vi "FPGA tester.vi"(4 "error in":errorcluster, 6 "Repetitions":dbl=1.0, 7 "Levels":i16[](array[numeric])) -> (0 "Error out":errorcluster[][](array[cluster]), 3 "Results":dbl[][](array[numeric]))   [LabVIEW 2013]
uses:
  <vilib>/DAQmx/read.llb/DAQmx Read (Counter DBL 1Chan 1Samp).vi
  <vilib>/DAQmx/write.llb/DAQmx Write (Digital Bool 1Line 1Point).vi
  <vilib>/DAQmx/read.llb/DAQmx Read (Digital Bool 1Line 1Point).vi
  <vilib>/Utility/file.llb/Read From Spreadsheet File (I64).vi
  <vilib>/DAQmx/create/channels.llb/DAQmx Create Channel (CI-Pulse Width).vi
  <vilib>/DAQmx/miscellaneous.llb/DAQmx Fill In Error Info.vi
  <vilib>/Utility/file.llb/Write To Spreadsheet File (DBL).vi
  <resource>/objmgr/daqmx.rc
panel:
  in  "Delay":u32
  in  "GPIB address":string="15"
  in  "Write to file?":bool
  out "Trial time vs. photons counted":cluster{"Y":dbl[], "Y":dbl[]}[](graph)
  out "all rows":i64[][](array[numeric])
  in  "Read Excel file?":bool
  out "Current level":u16
  out "Set 1":bool[](array[boolean])
  out "Set 2":bool[](array[boolean])
  out "Set 3":bool[](array[boolean])
  out "Set 4":bool[](array[boolean])
  out "16-bit number":bool[](array[boolean])
  # "Or specify levels below:"
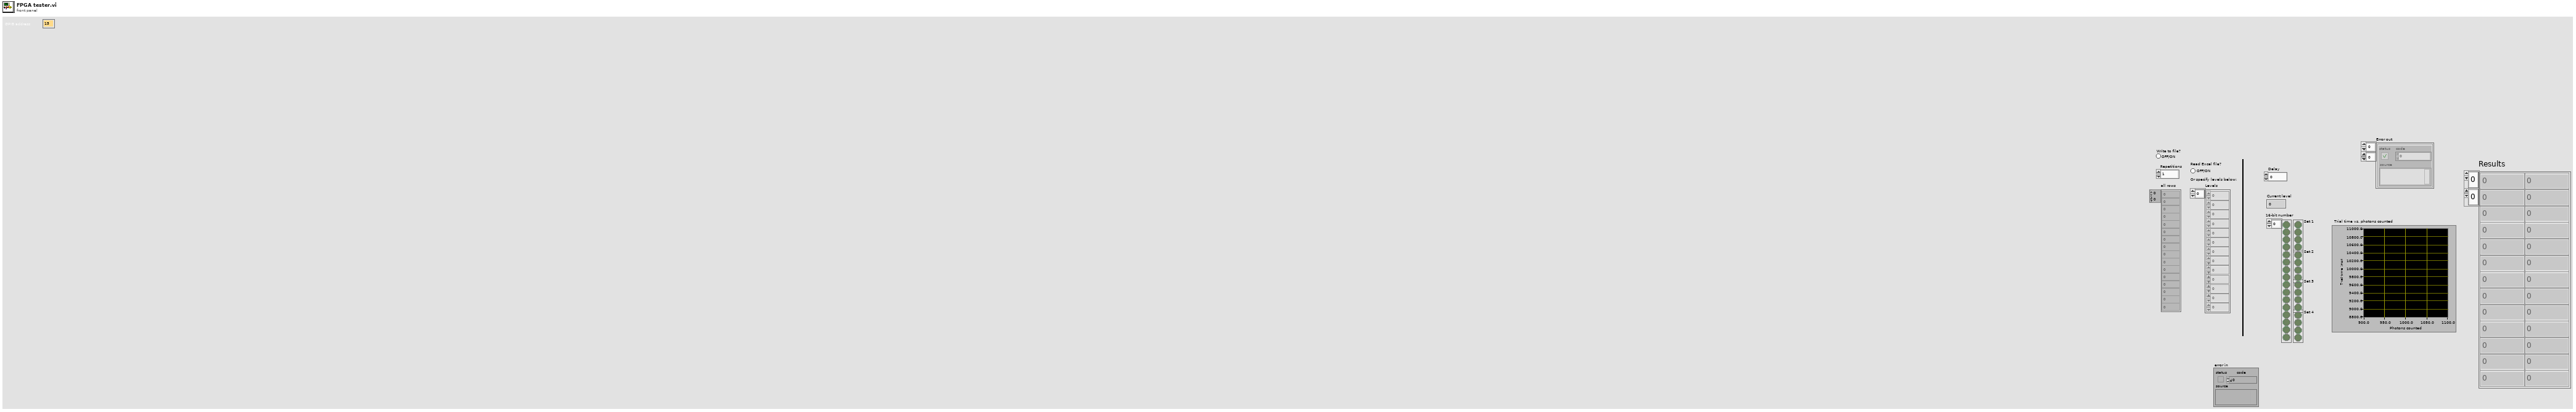
[diagram p1: front panel]
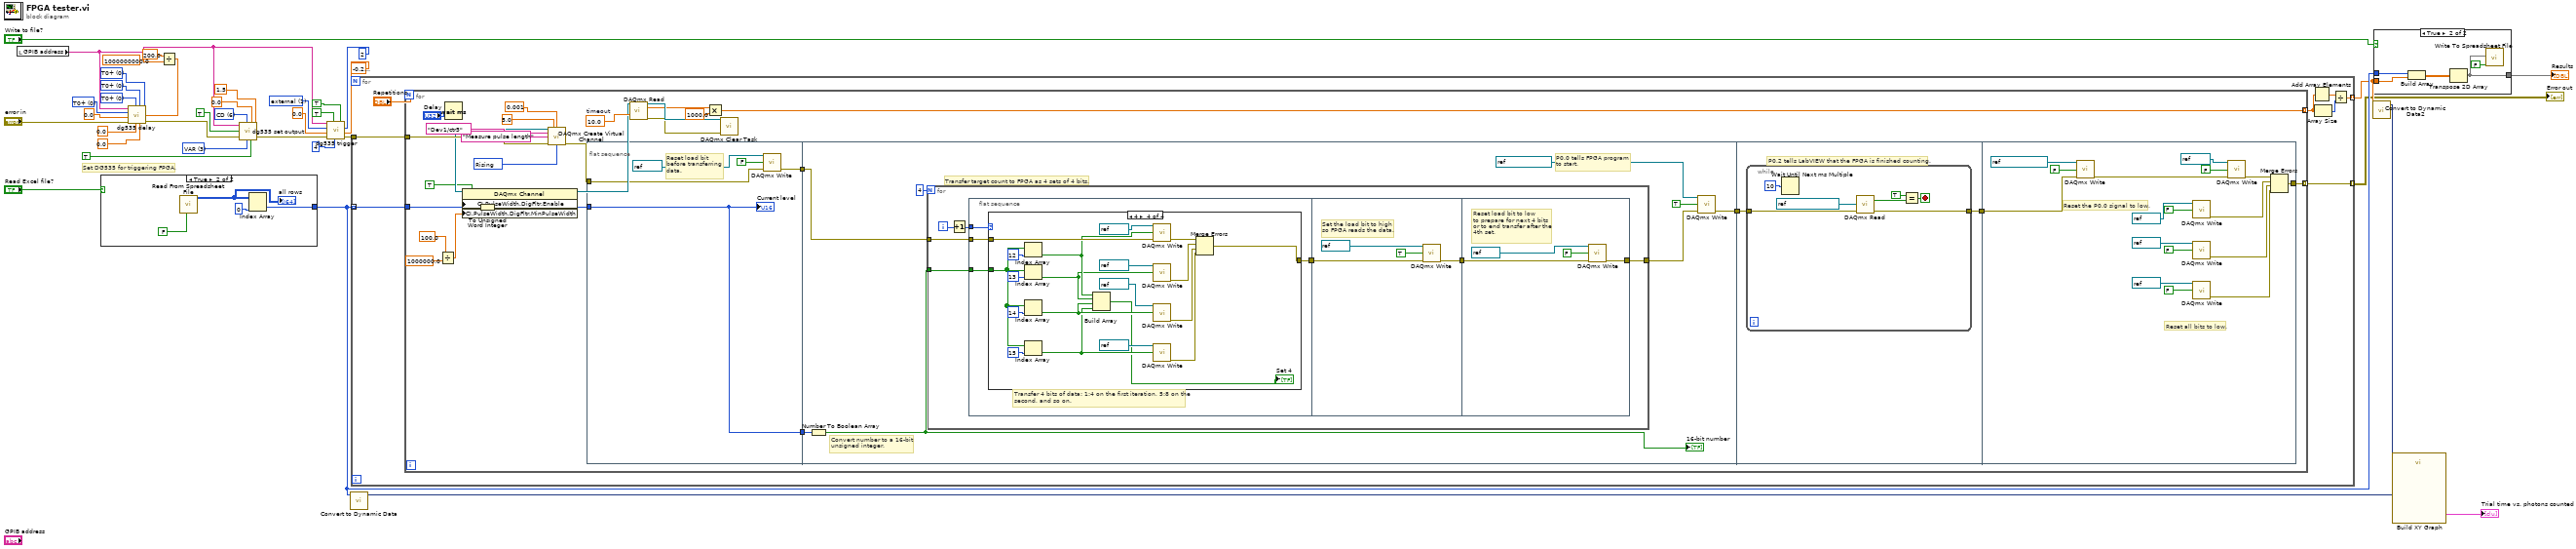
[diagram p0: block diagram]
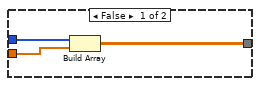
[diagram p2: hidden frame]
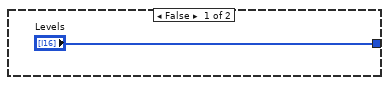
[diagram p3: hidden frame]
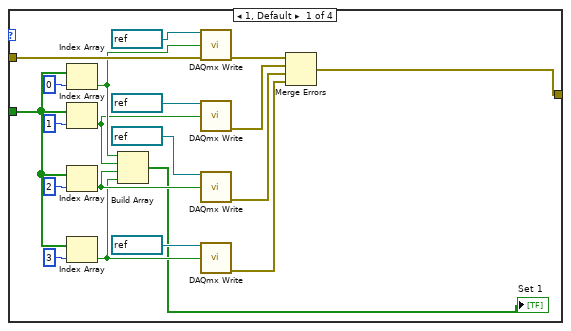
[diagram p4: hidden frame]
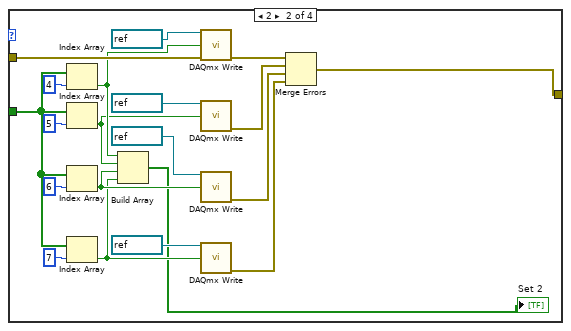
[diagram p5: hidden frame]
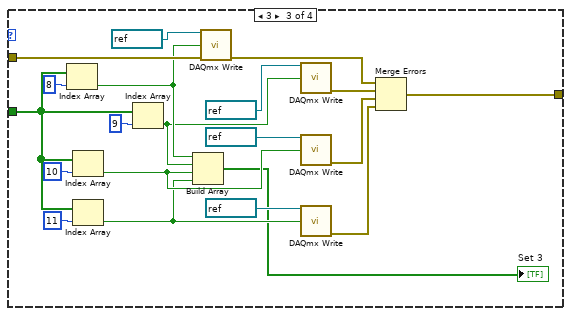
[diagram p6: hidden frame]
diagram:
  w18 = u32 1 items=["internal", "external", "single shot", "burst", "line"] ("trigger")
  w20 = 3 items=["TTL", "NIM", "ECL", "VAR"] ("mode")
  w22 = u16 6 items=["T0", "A", "B", "AB", "C", "D", "CD"] ("output")
  w25 = u32 0 items=["T0+", "A+", "B+", "C+"] ("D=")
  w26 = u32 0 items=["T0+", "A+", "B+", "D+"] ("C=")
  w27 = u32 0 items=["T0+", "A+", "C+", "D+"] ("B=")
  w28 = u32 0 items=["T0+", "B+", "C+", "D+"] ("A=")
  # "Set DG535 for triggering FPGA."
  n1 = local read "GPIB address"() -> (w10:string)
  n2 = case shown="True" "Read Excel file?" {
    tunnel: ["Levels" w41] -> w35
    frame False {
    }
    frame True {
      n3 = call-poly <vilib>:"Read From Spreadsheet File.vi"("transpose (no:F)"=FALSE) -> ("all rows"=w42:i64[][])  [unwired: 6 in, 4 out]
      "all rows" <- w42
      n4 = Index Array(array=w42, index (col)=0 ("disabled index (col)")) -> (element=w41:i64[])  [unwired: 1 in]
    }
  }
  n5 = Divide(x=200.0 ("D"), y=1000000000.0) -> (x/y=w4:dbl)
  n6 = call "dg535 delay.vi"("C"=0.0, "D"=w4, "D="=w25, "C="=w26, "B"=0.0 ("C"), "error in"="error in", "A"=0.0 ("D"), "B="=w27, "A="=w28, "GPIB address"=w10) -> ("error out"=w24:errorcluster)
  n7 = call "dg535 set output.vi"("GPIB address"=w10, "output"=w22, "set"=TRUE, "error in"=w24, "mode"=w20, "offset"=0.0, "amplitude"=1.5, "load"=TRUE) -> ("error out"=w11:errorcluster)  [unwired: 1 in]
  n8 = call "dg535 trigger.vi"("external trigger level"=sgl -0.2, "burst count"=2, "trigger slope"=TRUE, "burst period"=4, "input impedance"=TRUE, "error in"=w11, "internal/burst trigger rate"=0.0, "trigger"=w18, "GPIB address"=w10) -> ("error out"=w3:errorcluster)
  n9 = call "Convert to Dynamic Data"("Array"=w35) -> ("Dynamic Data Type"=w34:dynamicdata)  [unwired: 3 in]
  n10 = for {
    tunnel: w35 -> [w49] mode=indexing
    tunnel: [w45] -> w33 mode=indexing
    tunnel: w3 -> [w44]
    tunnel: [w43] -> w1 mode=indexing
    n11 = for {
      N: "Repetitions" -> [_]
      tunnel: w49 -> [w62]
      tunnel: [w61] -> w46 mode=indexing
      tunnel: w44 -> [w60]
      tunnel: [w58] -> w43 mode=indexing
      w66 = 10.0  # timeout
      w69 = 10280 items=["Rising"=10280, "Falling"=10171] ("Starting Edge")
      n12 = Divide(x=100.0 ("CI.PulseWidth.DigFltr.MinPulseWidth"), y=1000000.0) -> (x/y=w51:dbl)
      n13 = Wait (ms)(milliseconds to wait="Delay") -> ()  [unwired: 1 out]
      n14 = To Unsigned Word Integer(number=w62) -> (unsigned 16bit integer=w73:u16)
      n15 = call-poly <vilib>:"DAQmx Create Virtual Channel.vi"("maximum value"=5.0 ("Maximum Value (sec)"), "minimum value"=0.001 ("Minimum Value (sec)"), "counter"=tag "Dev1/ctr3" ("Physical Channel"), "name to assign"="Measure pulse length", "error in"=w60, "starting edge"=w69) -> ("task out"=w56:refnum<k21>, "error out"=w63:errorcluster)  [unwired: 8 in]
      n16 = property class="DAQmx Channel"(reference=w56, "CI.PulseWidth.DigFltr.Enable"=TRUE, "CI.PulseWidth.DigFltr.MinPulseWidth"=w51) -> (reference out=w55:refnum<k21>)  [unwired: 1 in, 1 out]
      n17 = flat-sequence {
        tunnel: w63 -> [w79]
        tunnel: w73 -> [w82]
        tunnel: [w82] -> w77
        tunnel: [w78] -> w76
        tunnel: [w83] -> w75
        tunnel: w77 -> [w90]
        tunnel: w76 -> [w87]
        tunnel: w75 -> [w191]
        tunnel: [w190] -> w74
        tunnel: [w199] -> w58
        tunnel: w74 -> [w205]
        frame #0 {
          # "Reset load bit\nbefore transferring\ndata."
          n18 = call-poly <vilib>:"DAQmx Write.vi"("task/channels in"=refnum<k21> "BIT5", "data"=FALSE, "error in"=w79) -> ("error out"=w78:errorcluster)  [unwired: 10 in, 2 out]
          "Current level" <- w82
        }
        frame #1 {
          # "P0.0 tells FPGA program \nto start."
          # "Convert number to a 16-bit\nunsigned integer."
          # "Transfer target count to FPGA as 4 sets of 4 bits."
          n19 = Number To Boolean Array(number=w90) -> (Boolean array=w88:bool[])
          "16-bit number" <- w88
          n20 = for {
            N: 4 -> [_]
            tunnel: w88 -> [w94]
            tunnel: w87 -> [w96]
            tunnel: [w91] -> w84
            i -> [w97]
            n21 = Increment(x=w97) -> (x+1=w95:i32)
            n22 = flat-sequence {
              tunnel: w96 -> [w101]
              tunnel: w95 -> [w100]
              tunnel: w94 -> [w99]
              tunnel: [w98] -> w93
              tunnel: w93 -> [w183]
              tunnel: [w182] -> w92
              tunnel: w92 -> [w187]
              tunnel: [w186] -> w91
              frame #0 {
                # "Transfer 4 bits of data: 1:4 on the first iteration, 5:8 on the\nsecond, and so on."
                n23 = case shown="4" w100 {
                  tunnel: w99 -> [w109 w129 w149 w169]
                  tunnel: w101 -> [w108 w128 w148 w168]
                  tunnel: [w107 w127 w147 w167] -> w98
                  frame 1, Default {
                    n24 = Index Array(array=w109, index=0) -> (element=w106:bool)
                    n25 = Index Array(array=w109, index=1) -> (element=w105:bool)
                    n26 = Index Array(array=w109, index=2) -> (element=w104:bool)
                    n27 = Index Array(array=w109, index=3) -> (element=w103:bool)
                    n28 = Build Array(w106, w105, w104, w103) -> (→"Set 1":bool[])
                    n29 = call-poly <vilib>:"DAQmx Write.vi"("task/channels in"=refnum<k21> "BIT1", "data"=w106, "error in"=w108) -> ("error out"=w117:errorcluster)  [unwired: 10 in, 2 out]
                    n30 = call-poly <vilib>:"DAQmx Write.vi"("task/channels in"=refnum<k21> "BIT2", "data"=w105) -> ("error out"=w116:errorcluster)  [unwired: 11 in, 2 out]
                    n31 = call-poly <vilib>:"DAQmx Write.vi"("task/channels in"=refnum<k21> "BIT3", "data"=w104) -> ("error out"=w115:errorcluster)  [unwired: 11 in, 2 out]
                    n32 = call-poly <vilib>:"DAQmx Write.vi"("task/channels in"=refnum<k21> "BIT4", "data"=w103) -> ("error out"=w114:errorcluster)  [unwired: 11 in, 2 out]
                    n33 = Merge Errors(w117, w116, w115, w114) -> (w107:errorcluster)
                  }
                  frame 2 {
                    n34 = Index Array(array=w129, index=4) -> (element=w126:bool)
                    n35 = Index Array(array=w129, index=5) -> (element=w125:bool)
                    n36 = Index Array(array=w129, index=6) -> (element=w124:bool)
                    n37 = Index Array(array=w129, index=7) -> (element=w123:bool)
                    n38 = Build Array(w126, w125, w124, w123) -> (→"Set 2":bool[])
                    n39 = call-poly <vilib>:"DAQmx Write.vi"("task/channels in"=refnum<k21> "BIT1", "data"=w126, "error in"=w128) -> ("error out"=w137:errorcluster)  [unwired: 10 in, 2 out]
                    n40 = call-poly <vilib>:"DAQmx Write.vi"("task/channels in"=refnum<k21> "BIT2", "data"=w125) -> ("error out"=w136:errorcluster)  [unwired: 11 in, 2 out]
                    n41 = call-poly <vilib>:"DAQmx Write.vi"("task/channels in"=refnum<k21> "BIT3", "data"=w124) -> ("error out"=w135:errorcluster)  [unwired: 11 in, 2 out]
                    n42 = call-poly <vilib>:"DAQmx Write.vi"("task/channels in"=refnum<k21> "BIT4", "data"=w123) -> ("error out"=w134:errorcluster)  [unwired: 11 in, 2 out]
                    n43 = Merge Errors(w137, w136, w135, w134) -> (w127:errorcluster)
                  }
                  frame 3 {
                    n44 = Index Array(array=w149, index=8) -> (element=w146:bool)
                    n45 = Index Array(array=w149, index=10) -> (element=w144:bool)
                    n46 = Index Array(array=w149, index=11) -> (element=w143:bool)
                    n47 = Index Array(array=w149, index=9) -> (element=w145:bool)
                    n48 = Build Array(w146, w145, w144, w143) -> (→"Set 3":bool[])
                    n49 = call-poly <vilib>:"DAQmx Write.vi"("task/channels in"=refnum<k21> "BIT1", "data"=w146, "error in"=w148) -> ("error out"=w157:errorcluster)  [unwired: 10 in, 2 out]
                    n50 = call-poly <vilib>:"DAQmx Write.vi"("task/channels in"=refnum<k21> "BIT2", "data"=w145) -> ("error out"=w156:errorcluster)  [unwired: 11 in, 2 out]
                    n51 = call-poly <vilib>:"DAQmx Write.vi"("task/channels in"=refnum<k21> "BIT3", "data"=w144) -> ("error out"=w155:errorcluster)  [unwired: 11 in, 2 out]
                    n52 = call-poly <vilib>:"DAQmx Write.vi"("task/channels in"=refnum<k21> "BIT4", "data"=w143) -> ("error out"=w154:errorcluster)  [unwired: 11 in, 2 out]
                    n53 = Merge Errors(w157, w156, w155, w154) -> (w147:errorcluster)
                  }
                  frame 4 {
                    n54 = Index Array(array=w169, index=12) -> (element=w166:bool)
                    n55 = Index Array(array=w169, index=13) -> (element=w165:bool)
                    n56 = Index Array(array=w169, index=14) -> (element=w164:bool)
                    n57 = Index Array(array=w169, index=15) -> (element=w163:bool)
                    n58 = Build Array(w166, w165, w164, w163) -> (→"Set 4":bool[])
                    n59 = call-poly <vilib>:"DAQmx Write.vi"("task/channels in"=refnum<k21> "BIT1", "data"=w166, "error in"=w168) -> ("error out"=w177:errorcluster)  [unwired: 10 in, 2 out]
                    n60 = call-poly <vilib>:"DAQmx Write.vi"("task/channels in"=refnum<k21> "BIT2", "data"=w165) -> ("error out"=w176:errorcluster)  [unwired: 11 in, 2 out]
                    n61 = call-poly <vilib>:"DAQmx Write.vi"("task/channels in"=refnum<k21> "BIT3", "data"=w164) -> ("error out"=w175:errorcluster)  [unwired: 11 in, 2 out]
                    n62 = call-poly <vilib>:"DAQmx Write.vi"("task/channels in"=refnum<k21> "BIT4", "data"=w163) -> ("error out"=w174:errorcluster)  [unwired: 11 in, 2 out]
                    n63 = Merge Errors(w177, w176, w175, w174) -> (w167:errorcluster)
                  }
                }
              }
              frame #1 {
                # "Set the load bit to high\nso FPGA reads the data."
                n64 = call-poly <vilib>:"DAQmx Write.vi"("task/channels in"=refnum<k21> "BIT5", "data"=TRUE, "error in"=w183) -> ("error out"=w182:errorcluster)  [unwired: 10 in, 2 out]
              }
              frame #2 {
                # "Reset load bit to low\nto prepare for next 4 bits\nor to end transfer after the\n4th set."
                n65 = call-poly <vilib>:"DAQmx Write.vi"("task/channels in"=refnum<k21> "BIT5", "data"=FALSE, "error in"=w187) -> ("error out"=w186:errorcluster)  [unwired: 10 in, 2 out]
              }
            }
          }
          n66 = call-poly <vilib>:"DAQmx Write.vi"("task/channels in"=refnum<k21> "LaserChannel", "data"=TRUE, "error in"=w84) -> ("error out"=w83:errorcluster)  [unwired: 10 in, 2 out]
        }
        frame #2 {
          # "P0.2 tells LabVIEW that the FPGA is finished counting."
          n67 = while {
            tunnel: w191 -> [w198]
            tunnel: [w197] -> w190
            stop <- w194 stop-if-true
            n68 = Wait Until Next ms Multiple(millisecond multiple=u32 10) -> ()  [unwired: 1 out]
            n69 = call-poly <vilib>:"DAQmx Read.vi"("task/channels in"=refnum<k21> "P02countSignal", "error in"=w198) -> ("data"=w195:bool, "error out"=w197:errorcluster)  [unwired: 11 in, 1 out]
            n70 = Equal?(x=TRUE, y=w195) -> (x = y?=w194:bool)
          }
        }
        frame #3 {
          # "Reset all bits to low."
          # "Reset the P0.0 signal to low."
          n71 = call-poly <vilib>:"DAQmx Write.vi"("task/channels in"=refnum<k21> "LaserChannel", "data"=FALSE, "error in"=w205) -> ("error out"=w204:errorcluster)  [unwired: 10 in, 2 out]
          n72 = call-poly <vilib>:"DAQmx Write.vi"("task/channels in"=refnum<k21> "BIT2", "data"=FALSE) -> ("error out"=w212:errorcluster)  [unwired: 11 in, 2 out]
          n73 = call-poly <vilib>:"DAQmx Write.vi"("task/channels in"=refnum<k21> "BIT3", "data"=FALSE) -> ("error out"=w211:errorcluster)  [unwired: 11 in, 2 out]
          n74 = call-poly <vilib>:"DAQmx Write.vi"("task/channels in"=refnum<k21> "BIT4", "data"=FALSE) -> ("error out"=w210:errorcluster)  [unwired: 11 in, 2 out]
          n75 = call-poly <vilib>:"DAQmx Write.vi"("task/channels in"=refnum<k21> "BIT1", "data"=FALSE, "error in"=w204) -> ("error out"=w213:errorcluster)  [unwired: 10 in, 2 out]
          n76 = Merge Errors(w213, w212, w211, w210) -> (w199:errorcluster)
        }
      }
      n77 = call-poly <vilib>:"DAQmx Read.vi"("task/channels in"=w55, "timeout"=w66) -> ("task out"=w68:refnum<k21>, "data"=w64:dbl, "error out"=w67:errorcluster)  [unwired: 11 in]
      n78 = Multiply(x=w64, y=1000.0) -> (x*y=w61:dbl)
      n79 = call <vilib>:"DAQmx Clear Task.vi"("task in"=w68, "error in"=w67) -> ()  [unwired: 13 in, 1 out]
    }
    n80 = Add Array Elements(numeric array=w46) -> (sum=w48:dbl)
    n81 = Array Size(array=w46) -> (size(s)=w47:i32)
    n82 = Divide(x=w48, y=w47) -> (x/y=w45:dbl)
  }
  "Error out" <- w1
  n83 = call "Convert to Dynamic Data2"("Array"=w33) -> ("Dynamic Data Type"=w32:dynamicdata)  [unwired: 3 in]
  n84 = case shown="True" "Write to file?" {
    tunnel: w33 -> [w217 w223]
    tunnel: w35 -> [w218 w222]
    tunnel: [w216 w219] -> w30
    frame False {
      n85 = Build Array(w218, w217) -> (w216:dbl[][])
    }
    frame True {
      n86 = Build Array(w222, w223) -> (w220:dbl[][])
      n87 = Transpose 2D Array(2D array=w220) -> (transposed array=w219:dbl[][])
      n88 = call-poly <vilib>:"Write To Spreadsheet File.vi"("append to file? (new file:F)"=FALSE, "2D data"=w219) -> ()  [unwired: 6 in, 1 out]
    }
  }
  "Results" <- w30
  n89 = call "Build XY Graph"("Y Input"=w32, "X Input"=w34) -> ("XY Graph"=→"Trial time vs. photons counted":cluster{"Y":dbl[], "Y":dbl[]}[])  [unwired: 3 in, 6 out]
